vi "Test Broadcast Latest Message Contet Correct.vi"(8 "error in (no error)":errorcluster, 11 "Test Case In":refnum<class "Debugger Test.lvclass">) -> (0 "error out":errorcluster, 3 "Test Case Out":refnum<class "Debugger Test.lvclass">)   [LabVIEW 2020, in "Debugger Test.lvclass"]
uses:
  Debugger Test.lvclass
  C:/Program Files (x86)/National Instruments/LabVIEW 2020/vi.lib/Astemes/LUnit/Test Case.lvclass
  source/Debugger/Debugger.lvclass
  C:/Users/anton/Documents/GitHub/triarc-debugger/source/Process/Debug Process.lvclass
  source/Debug Data/Raw Debug Data.ctl
  source/Debug Data/Debug Data.lvclass
  source/Process/Debug Process.lvclass/Debug Process.ctl
  <vilib>/Astemes/LUnit/Test Case.lvclass/Test Case.ctl
  <vilib>/Astemes/LUnit/LUnit Assertion Result.lvclass/LUnit Assertion Result.ctl
  <vilib>/Astemes/LUnit/LUnit Test Case Result.lvclass/LUnit Test Case Result.ctl
  <vilib>/Astemes/LUnit/LUnit Method Result.lvclass/LUnit Method Result.ctl
  01074fa8-ee8a-411d-bc8b-fc92c4f90959.vi
  source/Process/Public/Lifecycle/Get Lifecycle State.vi
  source/Process/Private/SubVIs/Wait for finish.vi
  source/Process/Protected/Messaging/Enqueue Message.vi
  source/Process/Private/SubVIs/Set Lifecycle State.vi
  <vilib>/Astemes/LUnit/Palette/Pass.vi
  <vilib>/Astemes/LUnit/Palette/Fail.vi
  <vilib>/Astemes/LUnit/Compare Variants.vi
  <vilib>/Astemes/LUnit/Describe Comparison.vi
  <vilib>/Astemes/LUnit/Set Assertion Type.vi
  <vilib>/Utility/error.llb/Clear Errors.vi
  <vilib>/Astemes/LUnit/Add test result.vi
  <vilib>/Astemes/LUnit/LUnit Write Passed.vi
  <vilib>/Astemes/LUnit/LUnit Write Message.vi
  <vilib>/Astemes/LUnit/LUnit Write Description.vi
  <vilib>/Astemes/LUnit/Variant to string.vi
  <vilib>/Astemes/LUnit/LUnit Write Assertion Type.vi
  <vilib>/Astemes/LUnit/LUnit Record Assertion Result.vi
  <vilib>/Astemes/LUnit/LUnit Aggregate Assertion Results.vi
  <vilib>/Astemes/LUnit/Assertion Result/LUnit Read Status.vi
  <vilib>/Astemes/LUnit/LUnit Read Message.vi
  <vilib>/Astemes/LUnit/LUnit Read Description.vi
  <vilib>/Astemes/LUnit/Method Result/LUnit Merge Status.vi
  <vilib>/Astemes/LUnit/LUnit Concatenate result strings.vi
  <vilib>/Utility/error.llb/Error Cluster From Error Code.vi
  <vilib>/Utility/Data Type/Get Type Information.vi
  <vilib>/Utility/LVClass/Get LV Class Name.vi
  <vilib>/Astemes/LUnit/LUnit Assertion Result.lvclass
  source/Process/Debug Process.lvclass
  Debugger Test.lvclass/Debugger Test.ctl
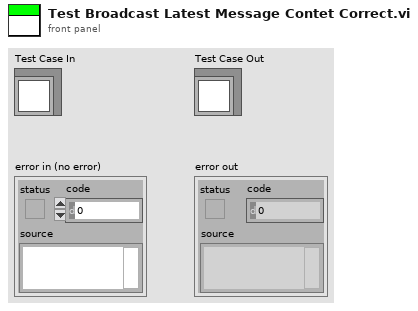
[diagram p1: front panel]
types:
  T1 = typedef "Debug Data.lvclass/Raw Debug Data.ctl" = cluster{"Action":string, "Call Chain":string, "Process":string, "Message":string, "Message Data":variant, "Time":dbl}
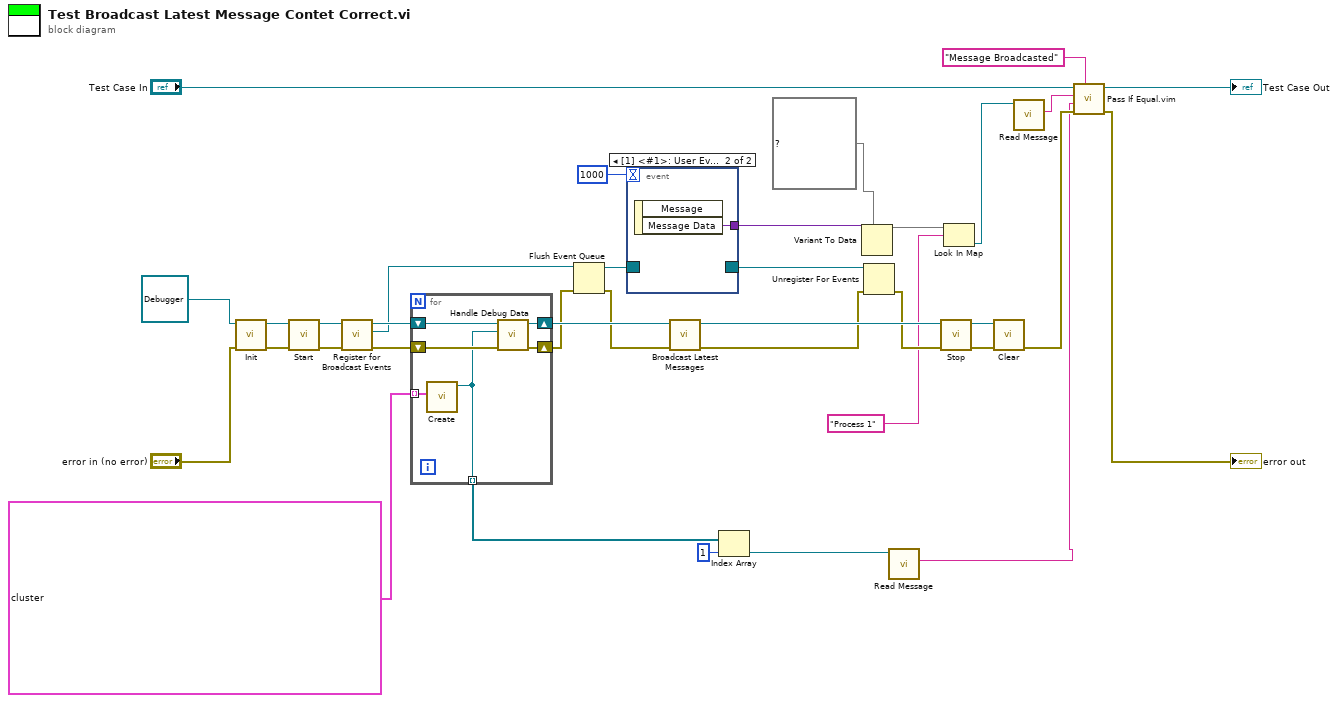
[diagram p0: block diagram]
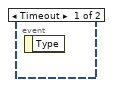
[diagram p2: hidden frame]
diagram:
  n1 = call-dynamic "Init.vi"("error in (no error)"="error in (no error)", "Process In"=refnum<class "Debugger.lvclass"> refnum ("Debug Data Event In 2")) -> ("error out"=w32:errorcluster, "Process Out"=w33:refnum<class "Debugger.lvclass">)  [unwired: 8 in]
  n2 = call "Start.vi"("error in (no error)"=w32, "Process In"=w33) -> ("error out"=w30:errorcluster, "Process Out"=w31:refnum<class "Debugger.lvclass">)  [unwired: 7 in, 1 out]
  n3 = call "Register for Broadcast Events.vi"("error in (no error)"=w30, "Process In"=w31) -> ("error out"=w29:errorcluster, "Event Registration Refnum Out"=w15:refnum<event-registration>, "Process Out"=w23:refnum<class "Debugger.lvclass">)  [unwired: 7 in]
  n4 = for {
    shift-right: [w40] -> w27
    shift-left: w29 -> [w42]
    shift-right: [w41] -> w28
    shift-left: w23 -> [w39]
    tunnel: T1[] [{"Action"="Send", "Call Chain"="Test.vi:123456", "Process"="Process 1", "Message"="Init", "Message Data"=variant, "Time"=0.0}, {"Action"="Receive", "Call Chain"="TF.lvlib:Process.lvclass:Handle Messages.vi:1960001", "Process"="Process 1", "Message"="Init", "Message Data"=variant, "Time"=0.0}, {"Action"="Send", "Call Chain"="Test.vi", "Process"="Process 1", "Message"="Start", "Message Data"=variant, "Time"=0.0}] ("Debug Data Cluster") -> [w38] mode=indexing
    tunnel: [w37] -> w3 mode=indexing
    n5 = call "Create.vi"("Debug Data Cluster"=w38) -> ("Debug Data out"=w37:refnum<class "Debug Data.lvclass">)  [unwired: 9 in, 1 out]
    n6 = call-dynamic "Handle Debug Data.vi"("error in (no error)"=w42, "Debug Data.lvclass"=w37, "Debug Data Event In"=w39) -> ("error out"=w40:errorcluster, "Debug Data Event Out"=w41:refnum<class "Debugger.lvclass">)  [unwired: 7 in]
  }
  n7 = Flush Event Queue(0:w15, 3:w27) -> (8:w14:refnum<event-registration>, 11:w16:errorcluster)  [unwired: 4 in, 1 out]
  n8 = event shown="[1] <#1>: User Event" {
    selector: w14 -> [_ _]
    dyn-events: [_ _] -> w18
    timeout: 1000 -> [_ _]
    tunnel: [_ w43] -> w11
    event Timeout {
      n9 = event-data() -> ()  [unwired: 1 in, 1 out]
    }
    event User Event {
      n10 = event-data() -> ("Message Data"=w43:variant)  [unwired: 1 in, 1 out]
    }
  }
  n11 = call "Broadcast Latest Messages.vi"("error in (no error)"=w16, "Debugger in"=w28) -> ("error out"=w13:errorcluster, "Debugger out"=w26:refnum<class "Debugger.lvclass">)  [unwired: 8 in]
  n12 = Index Array(array=w3, index=1) -> (element=w8:refnum<class "Debug Data.lvclass">)
  n13 = Variant To Data(type=map{string, refnum<class "Debug Data.lvclass">} {} ("Latest Messages"), Variant=w11) -> (data=w7:map{string, refnum<class "Debug Data.lvclass">})  [unwired: 1 in, 1 out]
  n14 = Unregister For Events(event registration refnum=w18, error in=w13) -> (error out=w12:errorcluster)
  n15 = call "Read Message.vi"("Debug Data in"=w8) -> ("Message"=w1:string)  [unwired: 8 in, 2 out]
  n16 = call "Stop.vi"("error in (no error)"=w12, "Process In"=w26) -> ("error out"=w24:errorcluster, "Process Out"=w25:refnum<class "Debugger.lvclass">)  [unwired: 7 in, 1 out]
  n17 = Look In Map(map=w7, key="Process 1") -> (value=w6:refnum<class "Debug Data.lvclass">)  [unwired: 1 in, 1 out]
  n18 = call-dynamic "Clear.vi"("error in (no error)"=w24, "Process In"=w25) -> ("error out"=w20:errorcluster)  [unwired: 9 in]
  n19 = call "Read Message.vi"("Debug Data in"=w6) -> ("Message"=w2:string)  [unwired: 8 in, 2 out]
  n20 = call "Pass If Equal.vim"("Description"="Message Broadcasted", "error in (no error)"=w20, "Actual"=w1, "Expected"=w2, "LUnit Test Case In"="Test Case In") -> ("error out"=→"error out":errorcluster, "LUnit Test Case Out"=→"Test Case Out":refnum<class "Debugger Test.lvclass">)  [unwired: 5 in]
